vi "ackAcceptCMD.vi"(8 "error in (no error)":errorcluster, 10 "CommandValue":T1=enum."disable", 11 "Model in":refnum<class "Model.lvclass">) -> (0 "error out":errorcluster, 3 "Model out":refnum<class "Model.lvclass">)   [LabVIEW 2016, in "Model.lvclass"]
uses:
  Model.lvclass
  Typedefs/CommandValue.ctl
  Model.lvclass/Model.ctl
  PubSubDataEvent/PubSubDataEvent.lvclass/PubSubDataEvent.ctl
  Typedefs/SEDSpectrometerTypedefs.lvlib
  PubSubDataEvent/PubSubDataEvent.lvclass
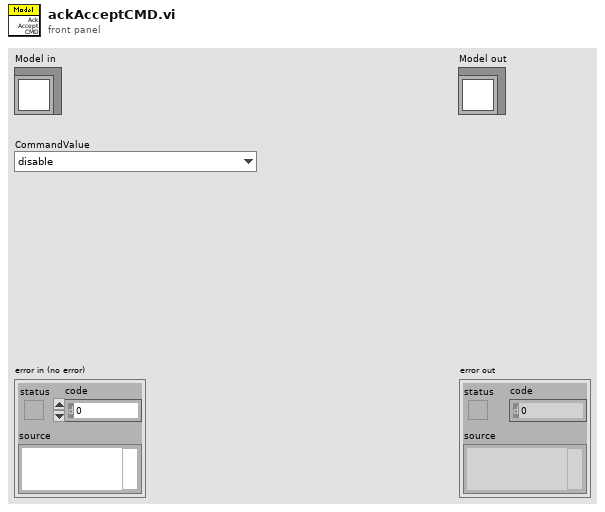
[diagram p1: front panel]
types:
  T1 = typedef "SEDSpectrometerTypedefs.lvlib/CommandValue.ctl" = enum16{"clearError", "disable", "enable", "exit", "GoToStandby", "OnHeartbeat", "OnIncomingMessagingError", "OnInterrupt", "start", "captureSpectImage", "setSpectTempSetpoint", "stopImageCapture"}
  T2 = cluster{"error":i32, "result":string, "ack":i32, "cmdSeqNum":i32, "CommandValue":T1}
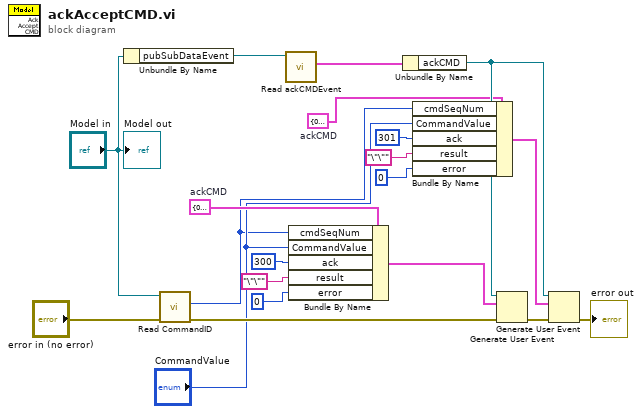
[diagram p0: block diagram]
diagram:
  w4 = T2 {"error"=0, "result"="", "ack"=0, "cmdSeqNum"=0, "CommandValue"=enum."disable"}  # ackCMD
  w13 = T2 {"error"=0, "result"="", "ack"=0, "cmdSeqNum"=0, "CommandValue"=enum."disable"}  # ackCMD
  n1 = Unbundle By Name("Model in") -> ("pubSubDataEvent"=w18:refnum<class "PubSubDataEvent.lvclass">)
  n2 = call-dynamic "Read CommandID.vi"("error in (no error)"="error in (no error)", "Model in"="Model in") -> ("error out"=w12:errorcluster, "CommandID"=w2:i32)  [unwired: 7 in, 1 out]
  n3 = call "Read ackCMDEvent.vi"("PubSubDataEvent in"=w18) -> ("ackCMDEvent"=w17:cluster{"ackCMD":refnum<user-event>})  [unwired: 8 in, 2 out]
  n4 = Bundle By Name(cluster=w13, "cmdSeqNum"=w2, "CommandValue"="CommandValue", "ack"=300, "result"="\"\"", "error"=0) -> (w11:T2)
  n5 = Unbundle By Name(w17) -> ("ackCMD"=w8:refnum<user-event>)
  n6 = Bundle By Name(cluster=w4, "cmdSeqNum"=w2, "CommandValue"="CommandValue", "ack"=301, "result"="\"\"", "error"=0) -> (w1:T2)
  n7 = Generate User Event(user event=w8, event data cluster=w11, error in=w12) -> (error out=w10:errorcluster)  [unwired: 1 in, 1 out]
  n8 = Generate User Event(user event=w8, event data cluster=w1, error in=w10) -> (error out=→"error out":errorcluster)  [unwired: 1 in, 1 out]
  "Model out" <- "Model in"
